vi "rad_Sort Software.vi"(8 "Analyzed Software 2":T1(array[cluster]), 9 "Different version":i32, 10 "Same version":i32, 11 "Analyzed Software 1":T1(array[cluster])) -> (0 "Sorted Software 2":string[](array[string]), 2 "Not matched":i32, 3 "Sorted Software 1":string[](array[string]))   [LabVIEW 2013]
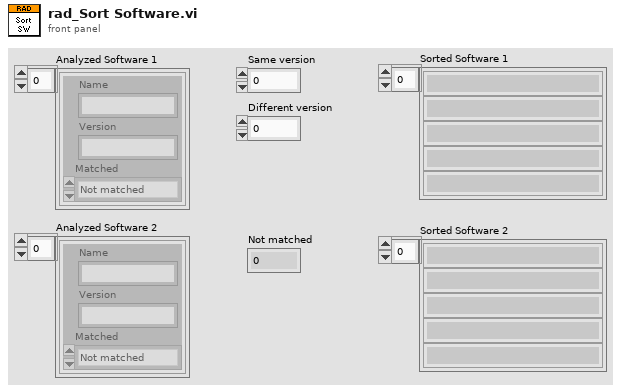
[diagram p1: front panel]
types:
  T1 = cluster{"Name":string, "Version":string, "Matched":enum16{"Not matched", "Different version", "Same version"}}[]
  T2 = enum16{"Not matched", "Different version", "Same version"}
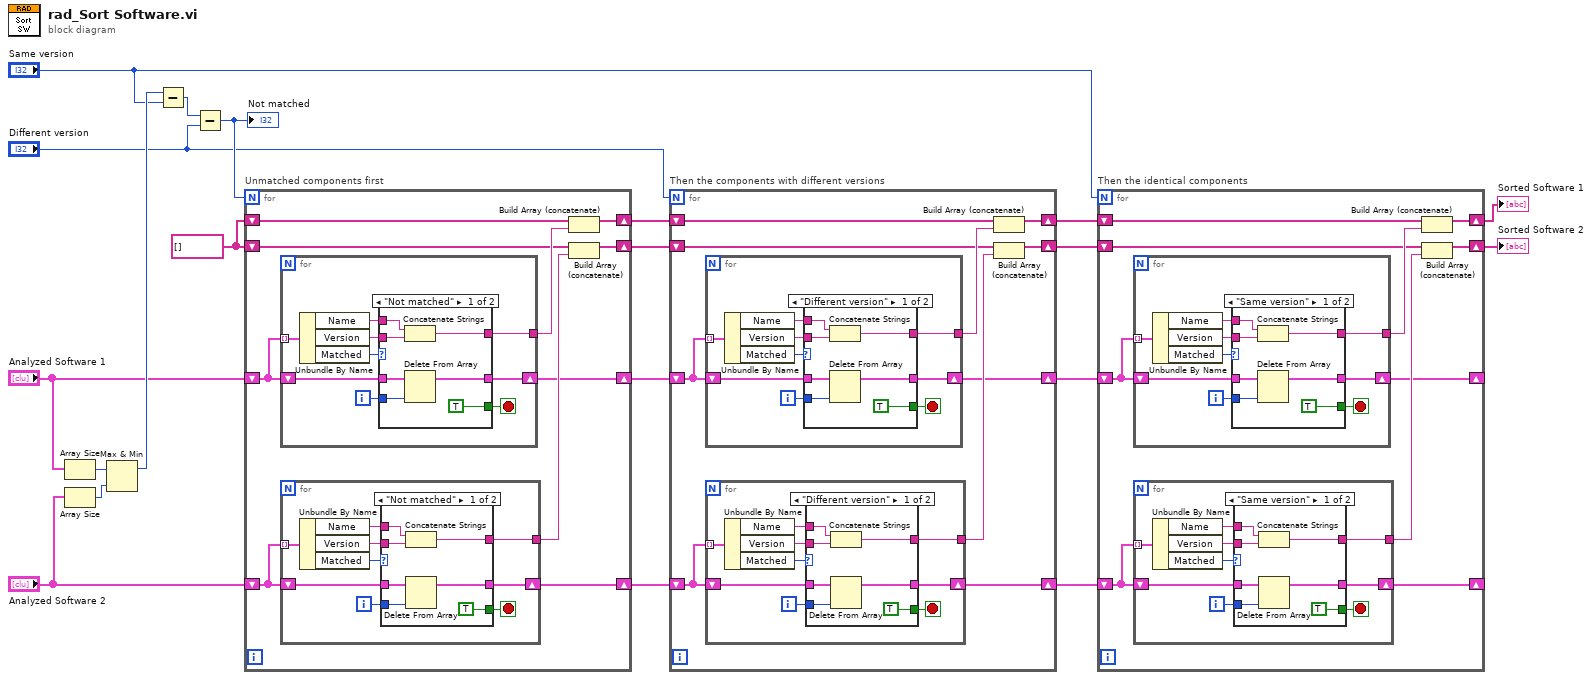
[diagram p0: block diagram]
diagram:
  w13 = string[] []
  n1 = Array Size(array="Analyzed Software 1") -> (size(s)=w20:i32)
  n2 = Array Size(array="Analyzed Software 2") -> (size(s)=w19:i32)
  n3 = Max & Min(x=w20, y=w19) -> (max(x,y)=w17:i32)  [unwired: 1 out]
  n4 = Subtract(x=w17, y="Same version") -> (x-y=w18:i32)
  n5 = Subtract(x=w18, y="Different version") -> (x-y=w16:i32)
  "Not matched" <- w16
  n6 = for "Unmatched components first" {
    N: w16 -> [_]
    shift-right: [w21] -> w10
    shift-left: "Analyzed Software 1" -> [w30]
    shift-right: [w26] -> w9
    shift-left: "Analyzed Software 2" -> [w22]
    shift-right: [w27] -> w12
    shift-left: w13 -> [w29]
    shift-right: [w23] -> w11
    shift-left: w13 -> [w25]
    n7 = for {
      shift-right: [w52] -> w21
      shift-left: w30 -> [w55]
      tunnel: w30 -> [w56] mode=indexing
      tunnel: [w49] -> w28
      i -> [w48]
      stop <- w53 stop-if-true
      n8 = Unbundle By Name(w56) -> ("Name"=w50:string, "Version"=w51:string, "Matched"=w54:T2)
      n9 = case shown="\"Not matched\"" w54 {
        tunnel: w55 -> [w59 w64]
        tunnel: [TRUE _] -> w53
        tunnel: [w57 w64] -> w52
        tunnel: w51 -> [w61 _]
        tunnel: w50 -> [w62 _]
        tunnel: [w60 _] -> w49
        tunnel: w48 -> [w58 _]
        frame "Not matched" {
          n10 = Concatenate Strings(w62, w61) -> (w60:string)
          n11 = Delete From Array(array=w59, index=w58) -> (array with subset deleted=w57:T1)  [unwired: 1 in, 1 out]
        }
        frame Default {
        }
      }
    }
    n12 = for {
      shift-right: [w35] -> w26
      shift-left: w22 -> [w38]
      tunnel: w22 -> [w39] mode=indexing
      tunnel: [w32] -> w24
      i -> [w31]
      stop <- w36 stop-if-true
      n13 = Unbundle By Name(w39) -> ("Name"=w33:string, "Version"=w34:string, "Matched"=w37:T2)
      n14 = case shown="\"Not matched\"" w37 {
        tunnel: w38 -> [w42 w47]
        tunnel: [TRUE _] -> w36
        tunnel: [w40 w47] -> w35
        tunnel: w34 -> [w44 _]
        tunnel: w33 -> [w45 _]
        tunnel: [w43 _] -> w32
        tunnel: w31 -> [w41 _]
        frame "Not matched" {
          n15 = Concatenate Strings(w45, w44) -> (w43:string)
          n16 = Delete From Array(array=w42, index=w41) -> (array with subset deleted=w40:T1)  [unwired: 1 in, 1 out]
        }
        frame Default {
        }
      }
    }
    n17 = Build Array (concatenate)(w29, w28) -> (w27:string[])
    n18 = Build Array (concatenate)(w25, w24) -> (w23:string[])
  }
  n19 = for "Then the components with different versions" {
    N: "Different version" -> [_]
    shift-right: [w65] -> w7
    shift-left: w10 -> [w74]
    shift-right: [w70] -> w8
    shift-left: w9 -> [w66]
    shift-right: [w71] -> w5
    shift-left: w12 -> [w73]
    shift-right: [w67] -> w6
    shift-left: w11 -> [w69]
    n20 = for {
      shift-right: [w96] -> w65
      shift-left: w74 -> [w99]
      tunnel: w74 -> [w100] mode=indexing
      tunnel: [w93] -> w72
      i -> [w92]
      stop <- w97 stop-if-true
      n21 = Unbundle By Name(w100) -> ("Name"=w94:string, "Version"=w95:string, "Matched"=w98:T2)
      n22 = case shown="\"Different version\"" w98 {
        tunnel: w99 -> [w103 w108]
        tunnel: [TRUE _] -> w97
        tunnel: [w101 w108] -> w96
        tunnel: w95 -> [w105 _]
        tunnel: w94 -> [w106 _]
        tunnel: [w104 _] -> w93
        tunnel: w92 -> [w102 _]
        frame "Different version" {
          n23 = Concatenate Strings(w106, w105) -> (w104:string)
          n24 = Delete From Array(array=w103, index=w102) -> (array with subset deleted=w101:T1)  [unwired: 1 in, 1 out]
        }
        frame Default {
        }
      }
    }
    n25 = for {
      shift-right: [w79] -> w70
      shift-left: w66 -> [w82]
      tunnel: w66 -> [w83] mode=indexing
      tunnel: [w76] -> w68
      i -> [w75]
      stop <- w80 stop-if-true
      n26 = Unbundle By Name(w83) -> ("Name"=w77:string, "Version"=w78:string, "Matched"=w81:T2)
      n27 = case shown="\"Different version\"" w81 {
        tunnel: w82 -> [w86 w91]
        tunnel: [TRUE _] -> w80
        tunnel: [w84 w91] -> w79
        tunnel: w78 -> [w88 _]
        tunnel: w77 -> [w89 _]
        tunnel: [w87 _] -> w76
        tunnel: w75 -> [w85 _]
        frame "Different version" {
          n28 = Concatenate Strings(w89, w88) -> (w87:string)
          n29 = Delete From Array(array=w86, index=w85) -> (array with subset deleted=w84:T1)  [unwired: 1 in, 1 out]
        }
        frame Default {
        }
      }
    }
    n30 = Build Array (concatenate)(w73, w72) -> (w71:string[])
    n31 = Build Array (concatenate)(w69, w68) -> (w67:string[])
  }
  n32 = for "Then the identical components" {
    N: "Same version" -> [_]
    shift-right: [w109] -> _
    shift-left: w7 -> [w118]
    shift-right: [w114] -> _
    shift-left: w8 -> [w110]
    shift-right: [w115] -> w4
    shift-left: w5 -> [w117]
    shift-right: [w111] -> w3
    shift-left: w6 -> [w113]
    n33 = for {
      shift-right: [w140] -> w109
      shift-left: w118 -> [w143]
      tunnel: w118 -> [w144] mode=indexing
      tunnel: [w137] -> w116
      i -> [w136]
      stop <- w141 stop-if-true
      n34 = Unbundle By Name(w144) -> ("Name"=w138:string, "Version"=w139:string, "Matched"=w142:T2)
      n35 = case shown="\"Same version\"" w142 {
        tunnel: w143 -> [w147 w152]
        tunnel: [TRUE _] -> w141
        tunnel: [w145 w152] -> w140
        tunnel: w139 -> [w149 _]
        tunnel: w138 -> [w150 _]
        tunnel: [w148 _] -> w137
        tunnel: w136 -> [w146 _]
        frame "Same version" {
          n36 = Concatenate Strings(w150, w149) -> (w148:string)
          n37 = Delete From Array(array=w147, index=w146) -> (array with subset deleted=w145:T1)  [unwired: 1 in, 1 out]
        }
        frame Default {
        }
      }
    }
    n38 = for {
      shift-right: [w123] -> w114
      shift-left: w110 -> [w126]
      tunnel: w110 -> [w127] mode=indexing
      tunnel: [w120] -> w112
      i -> [w119]
      stop <- w124 stop-if-true
      n39 = Unbundle By Name(w127) -> ("Name"=w121:string, "Version"=w122:string, "Matched"=w125:T2)
      n40 = case shown="\"Same version\"" w125 {
        tunnel: w126 -> [w130 w135]
        tunnel: [TRUE _] -> w124
        tunnel: [w128 w135] -> w123
        tunnel: w122 -> [w132 _]
        tunnel: w121 -> [w133 _]
        tunnel: [w131 _] -> w120
        tunnel: w119 -> [w129 _]
        frame "Same version" {
          n41 = Concatenate Strings(w133, w132) -> (w131:string)
          n42 = Delete From Array(array=w130, index=w129) -> (array with subset deleted=w128:T1)  [unwired: 1 in, 1 out]
        }
        frame Default {
        }
      }
    }
    n43 = Build Array (concatenate)(w117, w116) -> (w115:string[])
    n44 = Build Array (concatenate)(w113, w112) -> (w111:string[])
  }
  "Sorted Software 2" <- w3
  "Sorted Software 1" <- w4
